vi "Write Element by Index.vi"(8 "error in (no error)":errorcluster, 9 "MusicElement.lvclass":refnum<class "MusicElement.lvclass">, 10 "index":i32, 11 "MusicElementLibrary in":refnum<class "MusicElementLibrary.lvclass">) -> (0 "error out":errorcluster, 3 "MusicElementLibrary out":refnum<class "MusicElementLibrary.lvclass">, 5 "Written?":bool)   [LabVIEW 2015, in "MusicElementLibrary.lvclass"]
uses:
  MusicElementLibrary.lvclass
  MusicElement.lvclass
  MusicElementLibrary.lvclass/MusicElementLibrary.ctl
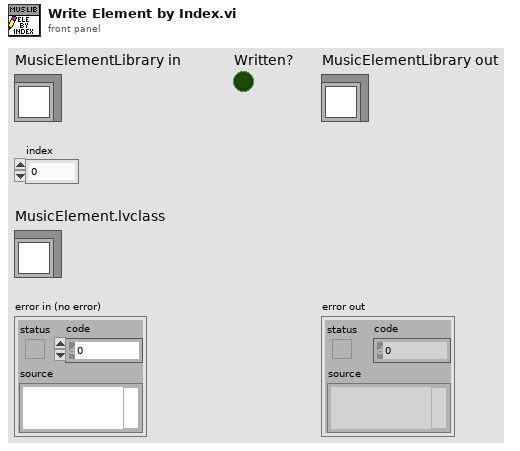
[diagram p1: front panel]
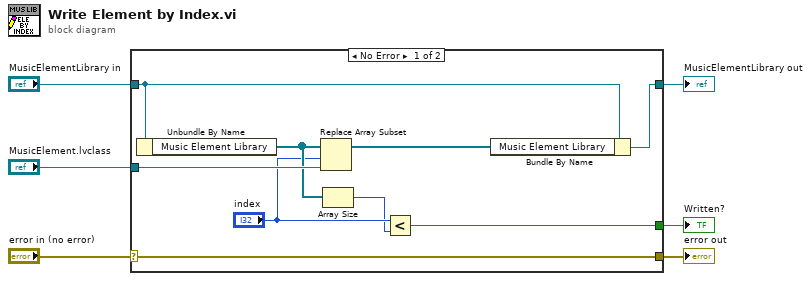
[diagram p0: block diagram]
diagram:
  n1 = case shown="No Error" "error in (no error)" {
    selector: "error in (no error)" -> [w15 w16]
    tunnel: [w15 w16] -> w5
    tunnel: [w14 w17] -> w3
    tunnel: "MusicElementLibrary in" -> [w13 w17]
    tunnel: "MusicElement.lvclass" -> [w11 _]
    tunnel: [w7 _] -> w1
    frame No Error {
      n2 = Unbundle By Name(w13) -> ("Music Element Library"=w10:refnum<class "MusicElement.lvclass">[])
      n3 = Replace Array Subset(array=w10, new element=w11, index="index") -> (w12:refnum<class "MusicElement.lvclass">[])
      n4 = Array Size(array=w10) -> (size(s)=w8:i32)
      n5 = Less?(x="index", y=w8) -> (x < y?=w7:bool)
      n6 = Bundle By Name(cluster=w13, "Music Element Library"=w12) -> (w14:refnum<class "MusicElementLibrary.lvclass">)
    }
    frame Error {
    }
  }
  "error out" <- w5
  "MusicElementLibrary out" <- w3
  "Written?" <- w1
